vi "Roller Loop.vi"   [LabVIEW 2013]
uses:
  Rollers/Roller Status.ctl
  Common Code/IR Logic State.ctl
  Robot Global Data.vi
  <vilib>/Rock Robotics/WPI/Solenoid/WPI_SolenoidSetEnum.vi
types:
  T1 = typedef "Roller Status.ctl" = cluster{"State":T2, "Front Power":dbl, "Front Solenoid":bool}
  T2 = typedef "IR Logic State.ctl" = enum16{"Waiting", "Requested", "Loading", "Full", "Wait for Center", "Carry", "Full Carry", "Holding"}
  T3 = typedef "WPI_SolenoidDevRef.ctl" = cluster{"DevStatus":errorcluster, "Solenoid Module":T4, "Forward Solenoid Channel":T5, "Reverse Solenoid Channel":T5}
  T4 = typedef "FPGA_TypedefSolenoidModule.ctl" = enum16{"Solenoid Module 1", "Solenoid Module 2"}
  T5 = typedef "WPI_SolenoidChannel.ctl" = enum8{"Solenoid 1", "Solenoid 2", "Solenoid 3", "Solenoid 4", "Solenoid 5", "Solenoid 6", "Solenoid 7", "Solenoid 8", "Invalid"}
  T6 = typedef "WPI_MotorControlDeviceRef.ctl" = cluster{"DeviceStatus":errorcluster, "Type":enum16{"PWM", "CAN"}, "PWM":cluster{"Digital Module":T7, "PWM Channel":T8, "DeadBand":T9}, "CAN":cluster{"Device Number":u8, "Control Mode":T10, "Semaphore":T11, "Max Vout":dbl}, "Invert":bool, "TransformRef":T12, "InvTransformRef":T12}
  T7 = typedef "FPGA_TypedefDigitalModule.ctl" = enum16{"Digital Module 1", "Digital Module 2"}
  T8 = typedef "FPGA_DIOPWMChannel.ctl" = enum8{"PWM 1", "PWM 2", "PWM 3", "PWM 4", "PWM 5", "PWM 6", "PWM 7", "PWM 8", "PWM 9", "PWM 10", "Invalid"}
  T9 = typedef "WPI_PWMDeadband.ctl" = cluster{"Name":string, "maxPositivePwm":i32, "minPositivePwm":i32, "centerPwm":i32, "maxNegativePwm":i32, "minNegativePwm":i32, "angularRange":u16}
  T10 = typedef "WPI_CANJaguar_ControlMode.ctl" = enum8{"Percent VBus", "Current", "Speed", "Position", "Voltage"}
  T11 = typedef "Semaphore RefNum" = refnum<k1>
  T12 = typedef "WPI_PWMTransform_ConPane.ctl" = refnum<vi>
  T13 = typedef "Roller Control.ctl" = cluster{"Mode":T14, "Front":enum16{"Stop", "Forward", "Reverse"}, "Back":enum16{"Stop", "Forward", "Reverse"}, "Reset":bool, "Front Piston":bool, "Halo":bool, "Net Piston":bool, "Carry Two":bool, "Hold":bool}
  T14 = typedef "Roller Mode.ctl" = enum16{"None", "Front", "Back", "Both", "Manual"}
  T15 = typedef "WPI_SolenoidValue.ctl" = enum16{"Off", "On", "Forward", "Reverse"}
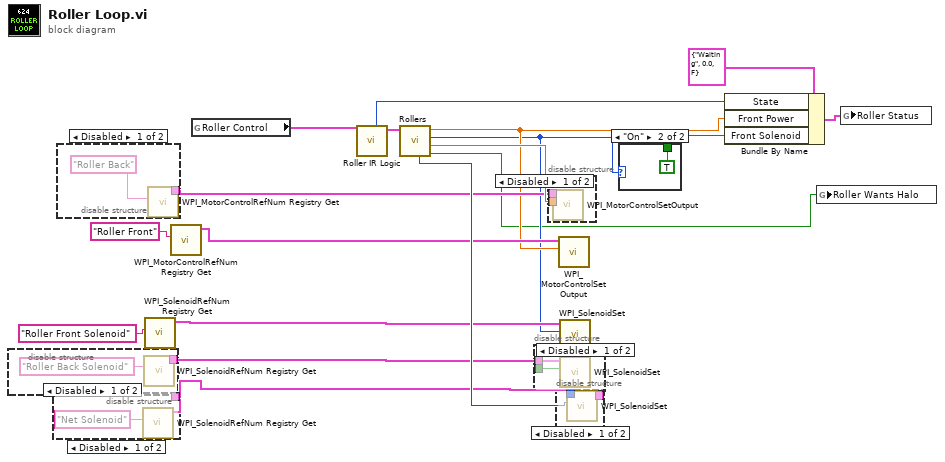
[diagram p0: block diagram]
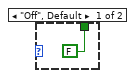
[diagram p8: hidden frame]
diagram:
  n1 = disable-structure shown="Disabled" {
    disable-tunnel: [w20 _] -> w11
    frame Disabled {
      n2 = call <vilib>:"WPI_SolenoidRefNum Registry Get.vi"("refnum name"="Roller Back Solenoid") -> ("SolenoidDevRef"=w20:T3)  [unwired: 9 in, 1 out]
    }
    frame Enabled {
    }
  }
  n3 = disable-structure shown="Disabled" {
    disable-tunnel: [w22 _] -> w10
    frame Disabled {
      n4 = call <vilib>:"WPI_SolenoidRefNum Registry Get.vi"("refnum name"="Net Solenoid") -> ("SolenoidDevRef"=w22:T3)  [unwired: 9 in, 1 out]
    }
    frame Enabled {
    }
  }
  n5 = disable-structure shown="Disabled" {
    disable-tunnel: [w23 _] -> w14
    frame Disabled {
      n6 = call <vilib>:"WPI_MotorControlRefNum Registry Get.vi"("refnum name"="Roller Back") -> ("MotorControlDevRef"=w23:T6)  [unwired: 9 in, 1 out]
    }
    frame Enabled {
    }
  }
  n7 = call <vilib>:"WPI_SolenoidRefNum Registry Get.vi"("refnum name"="Roller Front Solenoid") -> ("SolenoidDevRef"=w12:T3)  [unwired: 9 in, 1 out]
  n8 = call <vilib>:"WPI_MotorControlRefNum Registry Get.vi"("refnum name"="Roller Front") -> ("MotorControlDevRef"=w13:T6)  [unwired: 9 in, 1 out]
  n9 = global read "Robot Global Data.vi" "Roller Control"() -> (w9:T13)
  n10 = call "Roller IR Logic.vi"("Roller Command In"=w9) -> ("Roller Command Out"=w18:T13, "State"=w7:T2)  [unwired: 9 in]
  n11 = call "Rollers.vi"("Roller Command"=w18) -> ("Halo"=w1:bool, "Back Motor"=w16:dbl, "Front Solenoid"=w5:T15, "Front Motor"=w6:dbl, "Net Solenoid"=w17:T15)  [unwired: 6 in]
  n12 = disable-structure shown="Disabled" {
    disable-tunnel: _ -> [w26 _]
    disable-tunnel: w11 -> [w25 _]
    frame Disabled {
      n13 = call-poly <vilib>:"WPI_SolenoidSet.vi"("Value"=w26, "SolenoidDevRef"=w25) -> ()  [unwired: 8 in, 2 out]
    }
    frame Enabled {
    }
  }
  n14 = disable-structure shown="Disabled" {
    disable-tunnel: w16 -> [w28 _]
    disable-tunnel: w14 -> [w27 _]
    frame Disabled {
      n15 = call <vilib>:"WPI_MotorControlSetOutput.vi"("Output"=w28, "MotorControlDevRef"=w27) -> ()  [unwired: 7 in, 3 out]
    }
    frame Enabled {
    }
  }
  n16 = disable-structure shown="Disabled" {
    disable-tunnel: w10 -> [w31 _]
    disable-tunnel: [w30 _] -> _
    disable-tunnel: w17 -> [w29 _]
    frame Disabled {
      n17 = call-poly <vilib>:"WPI_SolenoidSet.vi"("Value"=w29, "SolenoidDevRef"=w31) -> ("SolenoidDevRef"=w30:T3)  [unwired: 8 in, 1 out]
    }
    frame Enabled {
    }
  }
  n18 = call <vilib>:"WPI_MotorControlSetOutput.vi"("Output"=w6, "MotorControlDevRef"=w13) -> ()  [unwired: 7 in, 3 out]
  n19 = call-poly <vilib>:"WPI_SolenoidSet.vi"("Value"=w5, "SolenoidDevRef"=w12) -> ()  [unwired: 8 in, 2 out]
  n20 = case shown="\"On\"" w5 {
    tunnel: [FALSE TRUE] -> w4
    frame "Off", Default {
    }
    frame "On" {
    }
  }
  n21 = Bundle By Name(cluster=T1 {"State"=enum."Waiting", "Front Power"=0.0, "Front Solenoid"=FALSE} ("Roller Status"), "State"=w7, "Front Power"=w6, "Front Solenoid"=w4) -> (w3:T1)
  n22 = global write "Robot Global Data.vi" "Roller Wants Halo"(w1) -> ()
  n23 = global write "Robot Global Data.vi" "Roller Status"(w3) -> ()
